vi "setSignalRateLimit.vi"(8 "error in":errorcluster, 9 "limit_Mcps":dbl, 10 "Slave Address (7-bit)":u8, 11 "I2C Ref In":T1) -> (0 "error out":errorcluster, 2 "Status":bool, 3 "I2C Ref Out":T1)   [LabVIEW 2018]
uses:
  <vilib>/myRIO/Instrument Drivers/Onboard IO/I2C/typedefs/I2C Reference.ctl
  <vilib>/myRIO/Common/Instrument Driver Framework/Utilities/typedefs/myRIO Generic Hardware Reference.ctl
  <vilib>/myRIO/Common/Instrument Driver Framework/Utilities/typedefs/Hardware Version Enum.ctl
  <vilib>/myRIO/Common/Instrument Driver Framework/Utilities/typedefs/myRIO v1.0 Reference.ctl
  <vilib>/myRIO/Common/Instrument Driver Framework/Utilities/typedefs/Generic FPGA Reference.ctl
  <vilib>/myRIO/Common/Instrument Driver Framework/myRIO v1.0/I2C/typedefs/I2C Channels Enum.ctl
  <vilib>/myRIO/Instrument Drivers/Onboard IO/I2C/typedefs/I2C Configuration.ctl
  <vilib>/myRIO/Instrument Drivers/Onboard IO/I2C/typedefs/I2C Transfer Rate.ctl
  <vilib>/Utility/error.llb/Error Cluster From Error Code.vi
  <vilib>/myRIO/Common/Instrument Driver Framework/myRIO v1.0/I2C/vis/myRIO v1.0 Write I2C.vi
  <vilib>/myRIO/Instrument Drivers/Onboard IO/I2C/I2C.lvlib
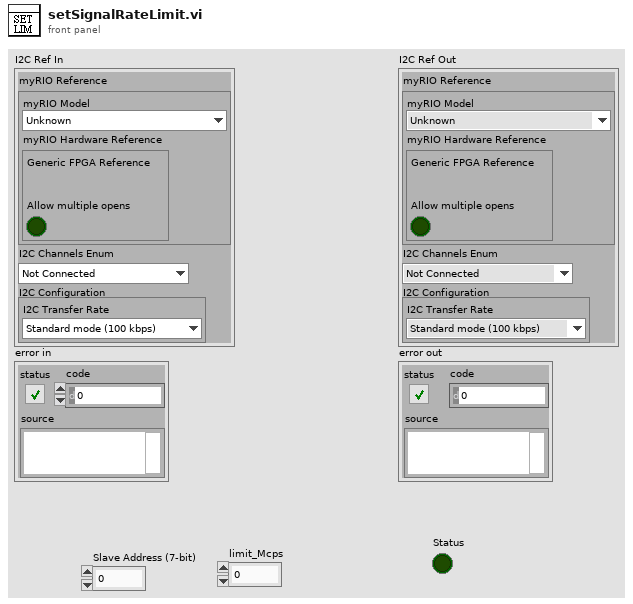
[diagram p1: front panel]
types:
  T1 = typedef "I2C.lvlib/I2C Reference.ctl" = cluster{"myRIO Reference":T2, "I2C Channels Enum":T6, "I2C Configuration":T7}
  T2 = typedef "myRIO Generic Hardware Reference.ctl" = cluster{"myRIO Model":T3, "myRIO Hardware Reference":T4}
  T3 = typedef "Hardware Version Enum.ctl" = enum16{"Unknown", "myRIO-1900", "myRIO-1950", "roboRIO", "NI ELVIS RIO CM", "ELVIS III"}
  T4 = typedef "myRIO v1.0 Reference.ctl" = cluster{"Generic FPGA Reference":T5, "Allow multiple opens":bool}
  T5 = typedef "Generic FPGA Reference.ctl" = refnum<k20>
  T6 = typedef "I2C Channels Enum.ctl" = enum16{"Not Connected", "A/I2C", "B/I2C", "I2C/I2C"}
  T7 = typedef "I2C.lvlib/I2C Configuration.ctl" = cluster{"I2C Transfer Rate":T8}
  T8 = typedef "I2C.lvlib/I2C Transfer Rate.ctl" = enum16{"Standard mode (100 kbps)", "Fast mode (400 kbps)"}
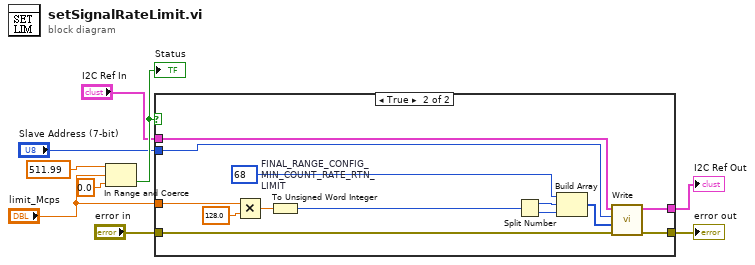
[diagram p0: block diagram]
diagram:
  n1 = In Range and Coerce(upper limit=511.99, x="limit_Mcps", lower limit=0.0) -> (In Range?=w9:bool)  [unwired: 1 out]
  "Status" <- w9
  n2 = case shown="True" w9 {
    tunnel: "limit_Mcps" -> [_ w22]
    tunnel: [w10 w16] -> w3
    tunnel: [w11 w15] -> w2
    tunnel: "Slave Address (7-bit)" -> [_ w14]
    tunnel: "error in" -> [w10 w13]
    tunnel: "I2C Ref In" -> [w11 w12]
    frame False {
    }
    frame True {
      w24 = u8 68  # FINAL_RANGE_CONFIG_MIN_COUNT_RATE_RTN_LIMIT
      n3 = Multiply(x=w22, y=128.0) -> (x*y=w20:dbl)
      n4 = To Unsigned Word Integer(number=w20) -> (unsigned 16bit integer=w19:u16)
      n5 = Split Number(x=w19) -> (hi(x)=w18:u8, lo(x)=w17:u8)
      n6 = Build Array(w24, w18, w17) -> (w23:u8[])
      n7 = call <vilib>:"Write.vi"("error in (no error)"=w13, "Bytes to Write"=w23, "Slave Address (7-bit)"=w14, "I2C Ref In"=w12) -> ("error out"=w16:errorcluster, "I2C Ref Out"=w15:T1)  [unwired: 6 in]
    }
  }
  "error out" <- w3
  "I2C Ref Out" <- w2
